vi "MissionOp Load Next.vi"(8 "error in (no error)":errorcluster, 11 "RDS Mission Controller Actor in":refnum<class "RDS Mission Controller Actor.lvclass">) -> (0 "error out":errorcluster, 3 "RDS Mission Controller Actor out":refnum<class "RDS Mission Controller Actor.lvclass">)   [LabVIEW 2015, in "RDS Mission Controller Actor.lvlib" / "RDS Mission Controller Actor.lvclass"]
uses:
  RDS Mission Controller Actor.lvclass
  RDS Mission Controller Actor.lvclass/RDS Mission Controller Actor.ctl
  Actors/RDS Controller Actor/RDS Controller Actor/Controller.ctl
  Libraries/RDS Child Messages/Controller Message/Controller Message Type.ctl
  Actors/RDS Controller Actor/RDS Controller Actor/RDS Controller Actor.lvlib
  Libraries/RDS Child Messages/Controller Message/Controller Message.lvclass
  Actors/RDS Parent Actor/RDS Parent Actor/RDS Parent Actor.lvclass
  Actors/RDS Helm Actor/RDS Helm Actor.lvlib
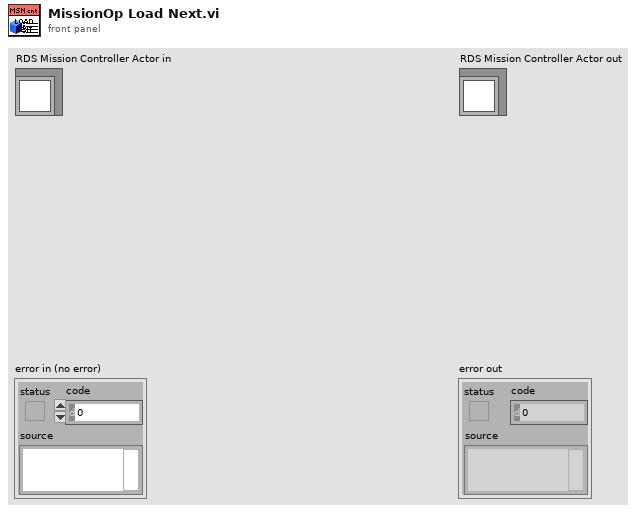
[diagram p1: front panel]
types:
  T1 = typedef "RDS Child Messages.lvlib/Controller Message.lvclass/Controller Message Type.ctl" = enum16{"Control Relinquish Request", "Control Relinquish Command", "Control Request", "Control Granted"}
  T2 = typedef "RDS Controller Actor.lvlib/Controller.ctl" = enum16{"Idle", "Local Remote Control", "Shore Remote Control", "Mission Control"}
  T3 = typedef "RDS Mission Controller Actor.lvlib/MissionOp.ctl" = cluster{"MissionOp Type":enum16{"Waypoint", "Loiter", "Wait", "Deploy AIP", "Stow AIP"}, "Duration (s)":u16, "Throttle":i16, "GPS Latitude":dbl, "GPS Longitude":dbl, "Loiter Range (m)":u16}
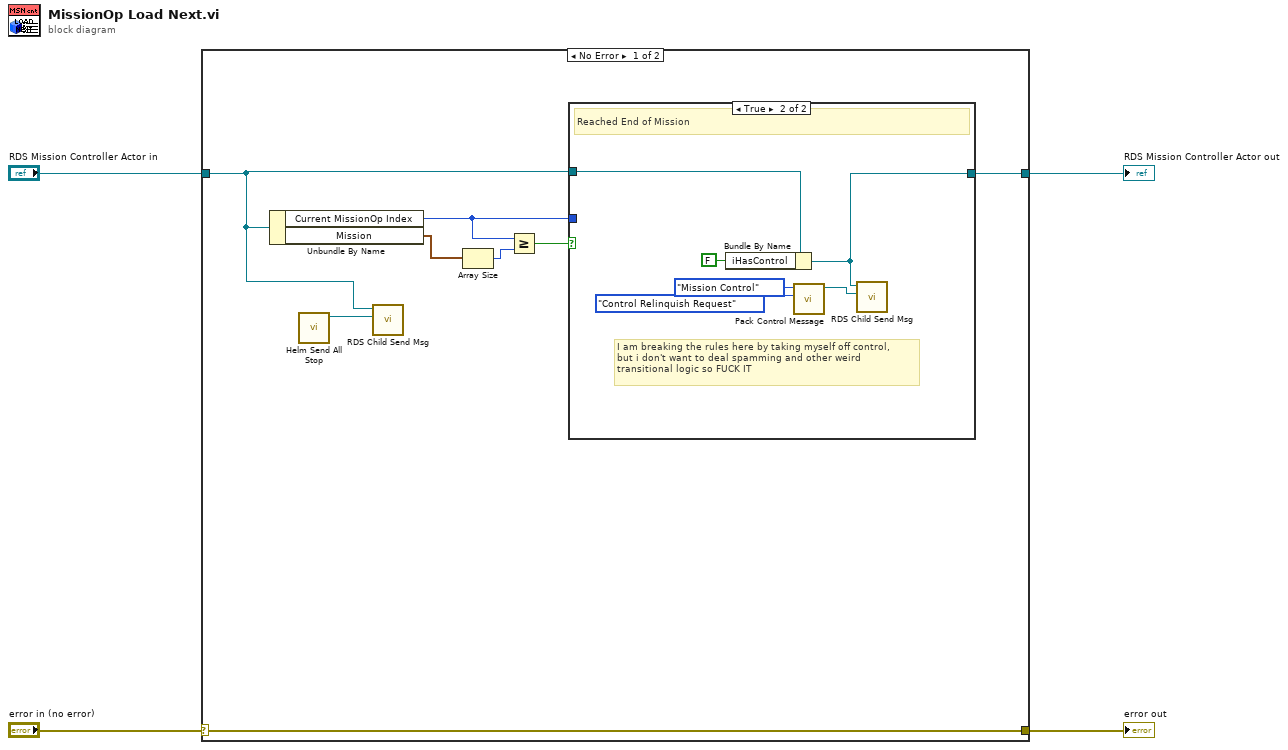
[diagram p0: block diagram]
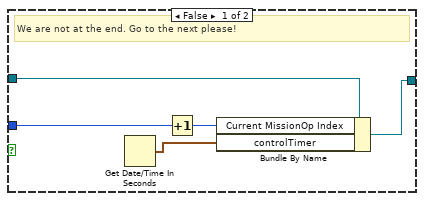
[diagram p2: hidden frame]
diagram:
  n1 = case shown="No Error" "error in (no error)" {
    selector: "error in (no error)" -> [w12 w25]
    tunnel: [w12 w25] -> w3
    tunnel: [w8 w24] -> w1
    tunnel: "RDS Mission Controller Actor in" -> [w5 w24]
    frame No Error {
      n2 = Unbundle By Name(w5) -> ("Current MissionOp Index"=w7:i32, "Mission"=w11:T3[])
      n3 = call "Helm Send All Stop.vi"() -> ("All Stop Message"=w6:refnum<class "Steering Command.lvclass">)  [unwired: 10 in, 1 out]
      n4 = call "RDS Child Send Msg.vi"("RDS Message"=w6, "RDS Parent Actor in"=w5) -> ()  [unwired: 8 in, 2 out]
      n5 = Array Size(array=w11) -> (size(s)=w10:i32)
      n6 = Greater Or Equal?(x=w7, y=w10) -> (x >= y?=w9:bool)
      n7 = case shown="True" w9 {
        tunnel: w5 -> [w17 w23]
        tunnel: [w16 w19] -> w8
        tunnel: w7 -> [w15 _]
        frame False {
          # "We are not at the end. Go to the next please!"
          n8 = Get Date/Time In Seconds() -> (seconds since 1Jan1904=w13:timestamp)
          n9 = Increment(x=w15) -> (x+1=w14:i32)
          n10 = Bundle By Name(cluster=w17, "Current MissionOp Index"=w14, "controlTimer"=w13) -> (w16:refnum<class "RDS Mission Controller Actor.lvclass">)
        }
        frame True {
          # "I am breaking the rules here by taking myself off control, \nbut i don't want to deal spamming and other weird \ntransitional logic so FUCK IT"
          # "Reached End of Mission"
          n11 = Bundle By Name(cluster=w23, "iHasControl"=FALSE) -> (w19:refnum<class "RDS Mission Controller Actor.lvclass">)
          n12 = call "Pack Control Message.vi"("Controller Message Type"=Controller_Message_Type."Control Relinquish Request", "Controller"=Controller."Mission Control") -> ("Controller Message out"=w18:refnum<class "Controller Message.lvclass">)  [unwired: 9 in]
          n13 = call "RDS Child Send Msg.vi"("RDS Message"=w18, "RDS Parent Actor in"=w19) -> ()  [unwired: 8 in, 2 out]
        }
      }
    }
    frame Error {
    }
  }
  "error out" <- w3
  "RDS Mission Controller Actor out" <- w1
